vi "WaitString.vi"(0 "reference":refnum<visa-resource-name>, 7 "String to Send":string, 11 "String to Receive":string) -> (4 "reference dup":refnum<visa-resource-name>, 8 "OK Done":bool, 15 "error out":errorcluster)   [LabVIEW 2019]
panel:
  # "Port Number 0=COM1"
  # "Send the 'String to Send' to the Stage Controller and wait for the 'String to Receive'.\nAn Error occurs when received a different string or timed out."
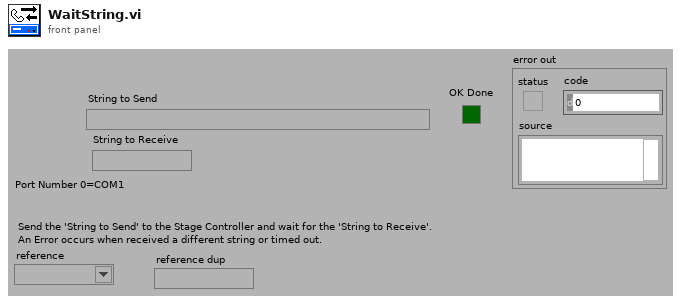
[diagram p1: front panel]
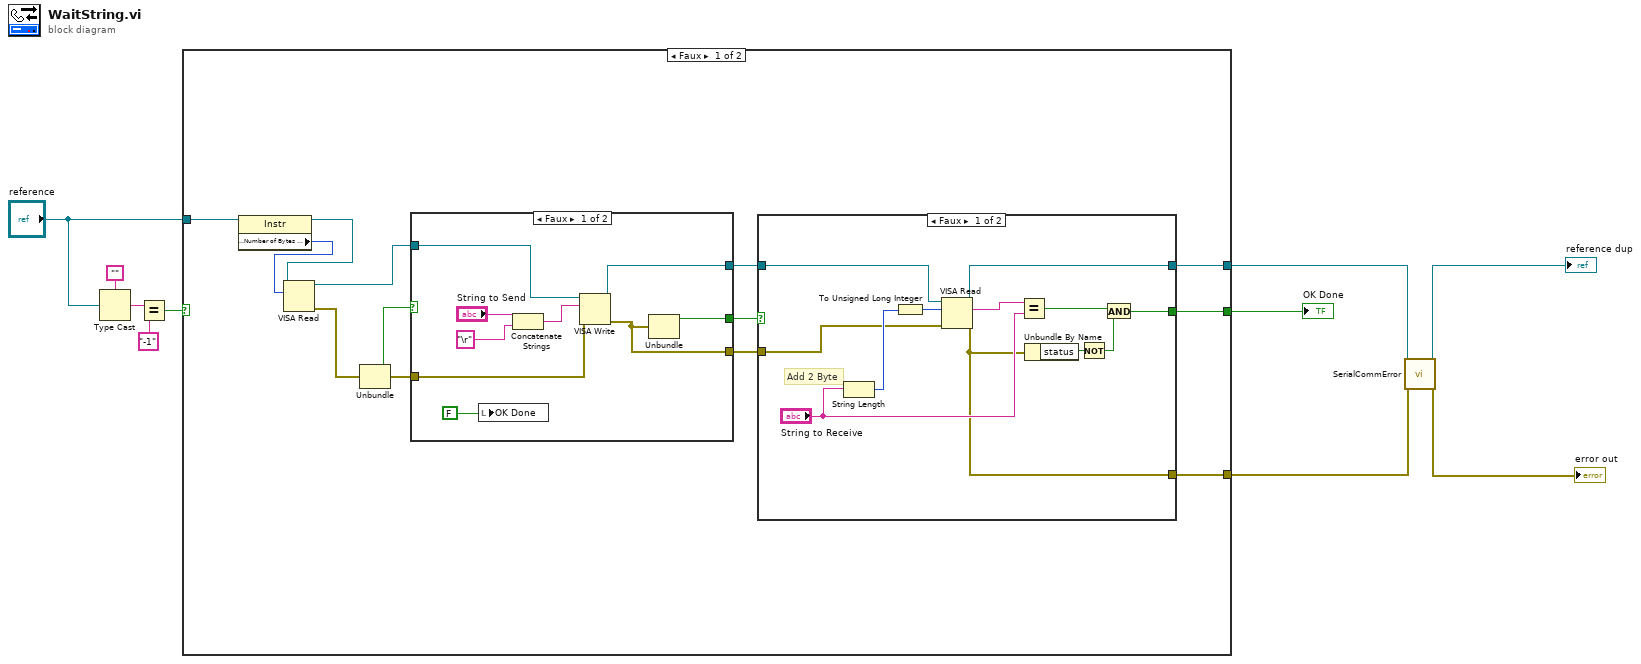
[diagram p0: block diagram]
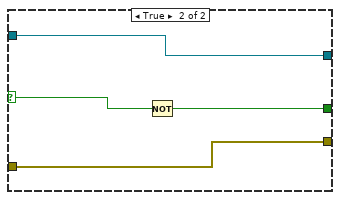
[diagram p2: hidden frame]
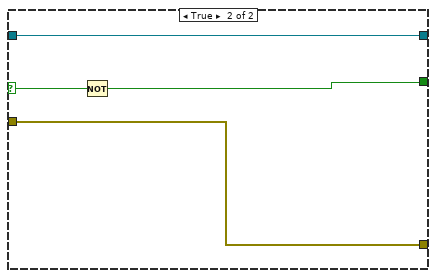
[diagram p3: hidden frame]
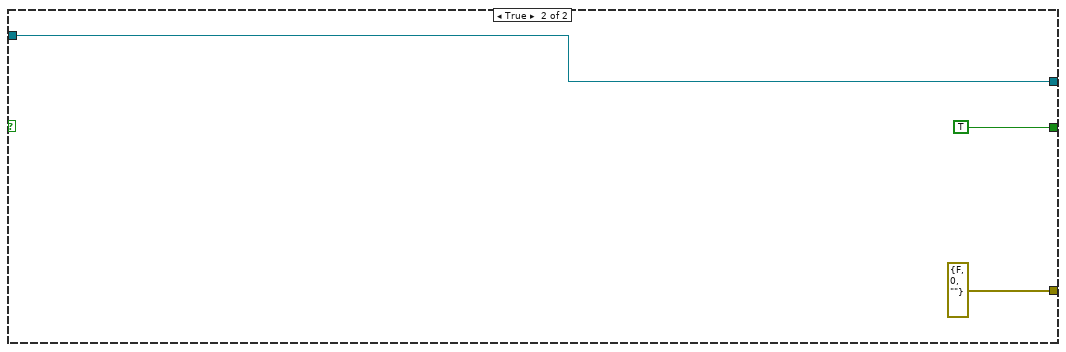
[diagram p4: hidden frame]
diagram:
  n1 = Type Cast(type="", x="reference") -> (*(type *) &x=w8:string)
  n2 = Equal?(x=w8, y="-1") -> (x = y?=w5:bool)
  n3 = case shown="Faux" w5 {
    tunnel: [w21 TRUE] -> w10
    tunnel: "reference" -> [w16 w52]
    tunnel: [w14 errorcluster {"status"=FALSE, "code"=0, "source"=""} ("error out")] -> w3
    tunnel: [w11 w52] -> w4
    frame False {
      n4 = property class="Instr"(reference=w16) -> (reference out=w19:refnum<visa-resource-name>, "Serial Settings:Number of Bytes at Serial Port"=w18:u32)  [unwired: 1 in, 1 out]
      n5 = VISA Read(VISA resource name=w19, byte count=w18) -> (VISA resource name out=w17:refnum<visa-resource-name>, error out=w12:errorcluster)  [unwired: 1 in, 2 out]
      n6 = Unbundle(w12) -> ("status"=w20:bool)  [unwired: 2 out]
      n7 = case shown="Faux" w20 {
        selector: w20 -> [_ w35]
        tunnel: [w25 w34] -> w22
        tunnel: [w27 w33] -> w15
        tunnel: w17 -> [w26 w33]
        tunnel: [w24 w32] -> w13
        tunnel: w12 -> [w23 w32]
        frame False {
          n8 = local write "OK Done"(FALSE) -> ()
          n9 = Concatenate Strings("String to Send", "\r") -> (w28:string)
          n10 = VISA Write(VISA resource name=w26, write buffer=w28, error in (no error)=w23) -> (VISA resource name out=w27:refnum<visa-resource-name>, error out=w24:errorcluster)  [unwired: 1 out]
          n11 = Unbundle(w24) -> ("status"=w25:bool)  [unwired: 2 out]
        }
        frame True {
          n12 = Not(x=w35) -> (.not. x?=w34:bool)
        }
      }
      n13 = case shown="Faux" w22 {
        selector: w22 -> [_ w51]
        tunnel: [w47 w50] -> w21
        tunnel: w15 -> [w37 w48]
        tunnel: [w39 w49] -> w14
        tunnel: w13 -> [w38 w49]
        tunnel: [w36 w48] -> w11
        frame False {
          # "Add 2 Byte"
          n14 = String Length(string="String to Receive") -> (length=w45:i32)
          n15 = To Unsigned Long Integer(number=w45) -> (unsigned 32bit integer=w40:u32)
          n16 = VISA Read(VISA resource name=w37, byte count=w40, error in (no error)=w38) -> (VISA resource name out=w36:refnum<visa-resource-name>, read buffer=w42:string, error out=w39:errorcluster)  [unwired: 1 out]
          n17 = Equal?(x=w42, y="String to Receive") -> (x = y?=w41:bool)
          n18 = Unbundle By Name(w39) -> ("status"=w44:bool)
          n19 = Not(x=w44) -> (.not. x?=w43:bool)
          n20 = And(x=w41, y=w43) -> (x .and. y?=w47:bool)
        }
        frame True {
          n21 = Not(x=w51) -> (.not. x?=w50:bool)
        }
      }
    }
    frame True {
    }
  }
  "OK Done" <- w10
  n22 = call "SerialCommError.vi"("VISA IN"=w4, "error IN"=w3) -> ("VISA OUT"=→"reference dup":refnum<visa-resource-name>, "error OUT"=→"error out":errorcluster)  [unwired: 11 in, 1 out]
